vi "test_TCP_TCP Write.vi"(8 "error in (no error)":errorcluster, 11 "TestCase in":refnum<class "Ethernet Protocol Tests.lvclass">) -> (0 "error out":errorcluster, 3 "TestCase out":refnum<class "Ethernet Protocol Tests.lvclass">)   [LabVIEW 2019, in "Ethernet Protocol Tests.lvclass"]
uses:
  Ethernet Protocol Tests.lvclass
  Listener/Listener.lvclass
  Listener/ListenerClassControls/Operation.ctl
  TCP/TCP.lvclass
  D:/GitRepository/niveristand-instrument-addon-classes/Source/Protocols/Protocol Parent/Protocol Parent.lvclass
  TCP/TCP.lvclass/TCP.ctl
  <vilib>/addons/_JKI Toolkits/VI Tester/TestCase.llb/TestCase.lvclass
  C:/Program Files (x86)/National Instruments/LabVIEW 2019/vi.lib/addons/_JKI Toolkits/VI Tester/TestCase.llb/TestCase.lvclass
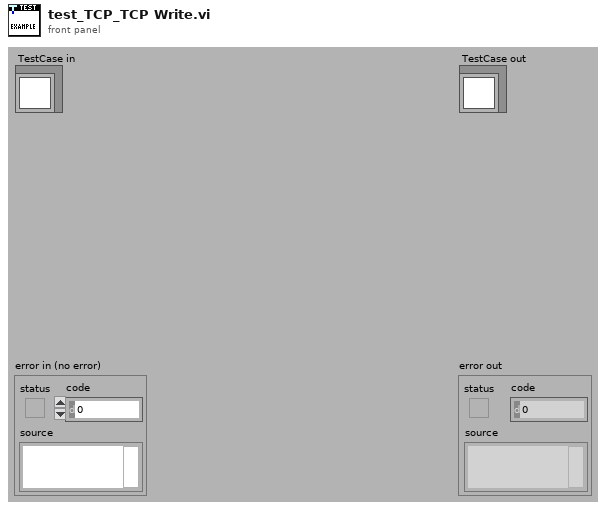
[diagram p1: front panel]
types:
  T1 = typedef "Listener.lvclass/Operation.ctl" = enum16{"Read", "Write"}
  T2 = typedef "Listener.lvclass/TCP Data Structure.ctl" = cluster{"TCP|IP connection ID":refnum<k5>, "IP Address":string, "Port":u16, "Data":string}
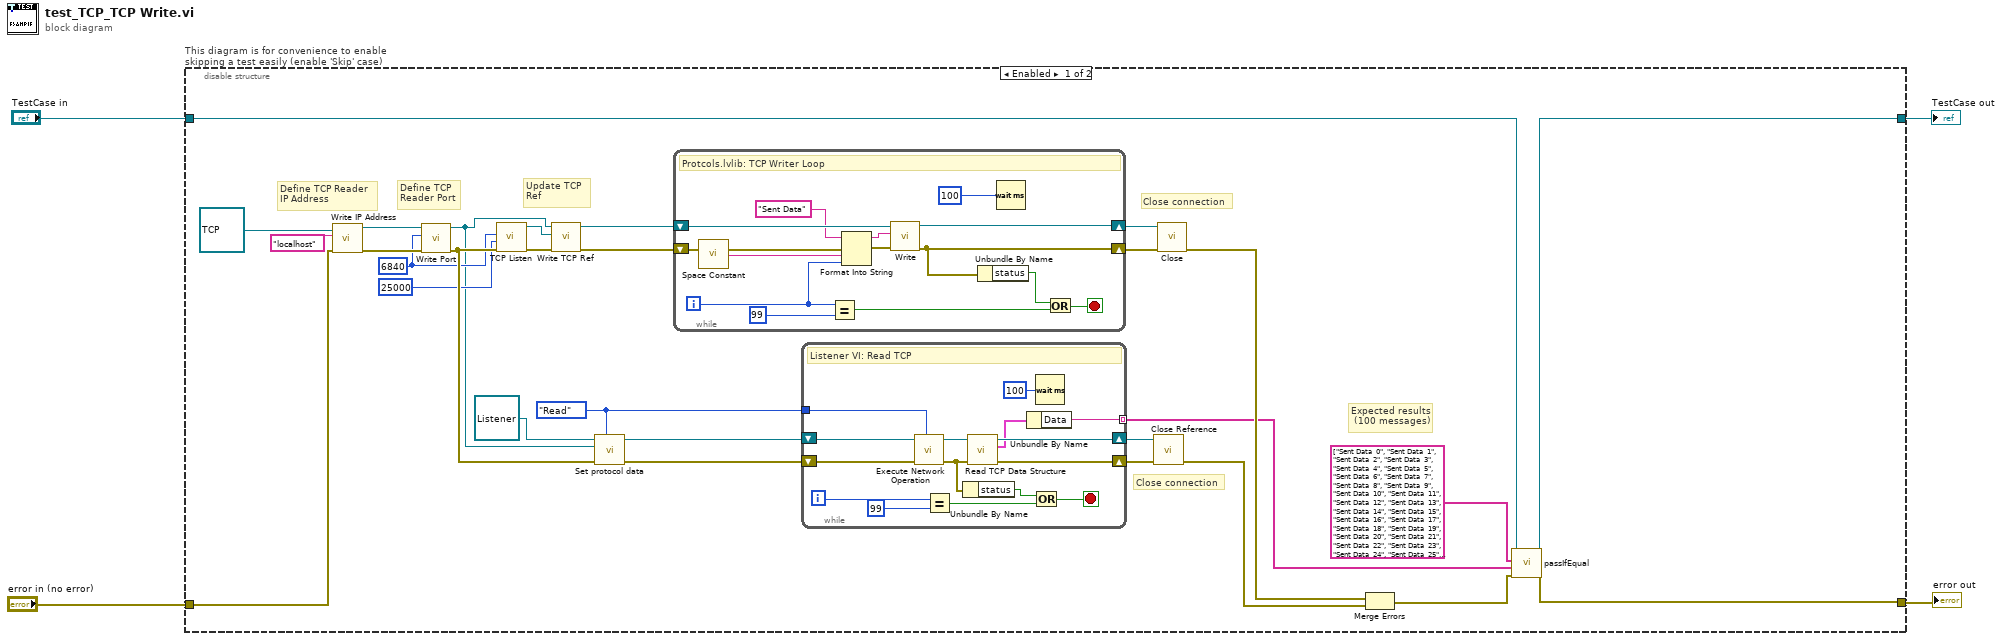
[diagram p0: block diagram]
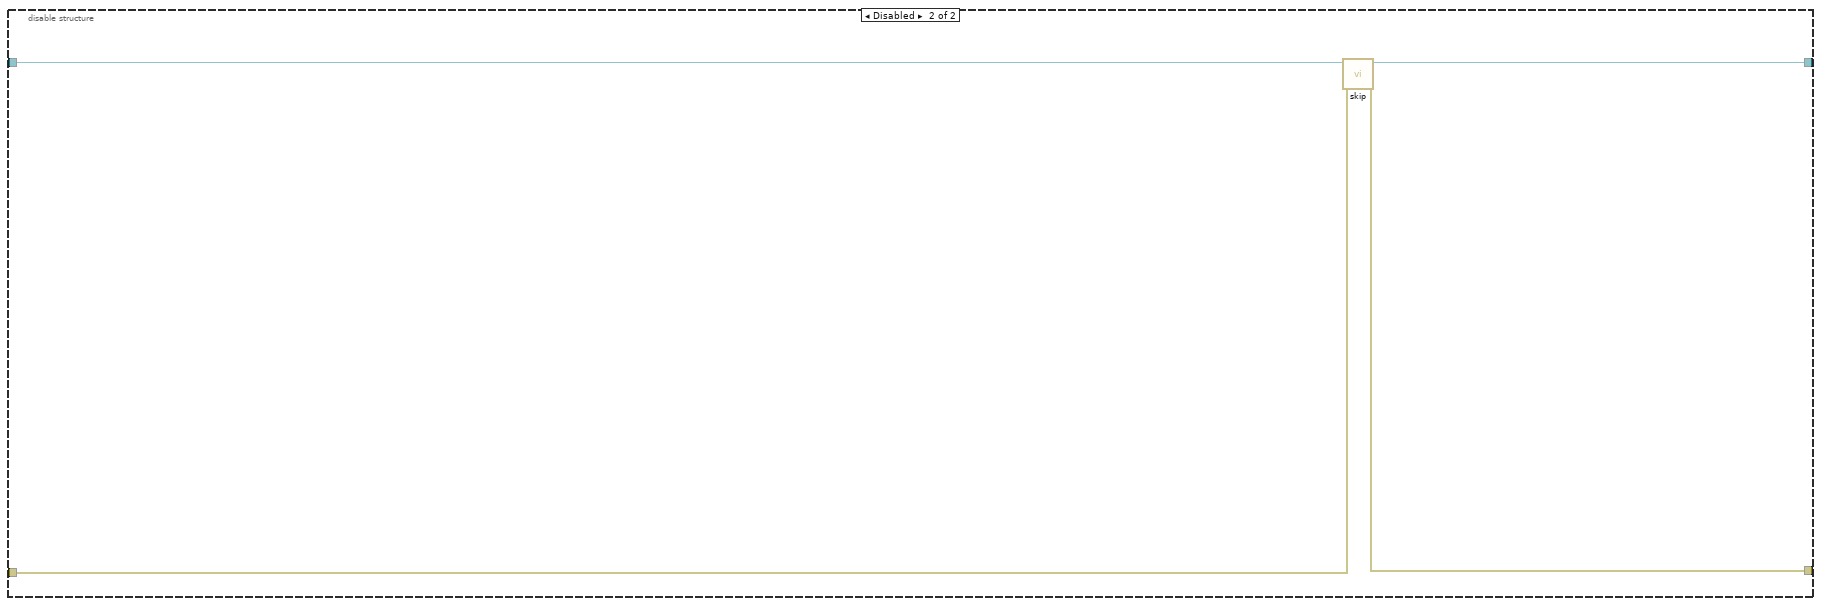
[diagram p2: hidden frame]
diagram:
  n1 = disable-structure "This diagram is for convenience to enable skipping a test easily (enable 'Skip' case)" shown="Enabled" {
    disable-tunnel: "TestCase in" -> [w33 w66]
    disable-tunnel: [w32 w64] -> w1
    disable-tunnel: [w31 w65] -> w3
    disable-tunnel: "error in (no error)" -> [w27 w63]
    frame Enabled {
      w14 = Operation."Read" ("Operation")
      w21 = u16 6840 ("Port")
      # "Close connection"
      # "Close connection"
      # "Update TCP \nRef"
      # "Expected results\n (100 messages)"
      # "Define TCP \nReader Port"
      # "Define TCP Reader \nIP Address"
      n2 = call "Write IP Address.vi"("error in (no error)"=w27, "IP Address"="localhost", "Ethernet in"=refnum<class "TCP.lvclass"> refnum ("Protocols.lvlib:TCP.lvclass")) -> ("error out"=w28:errorcluster, "Ethernet out"=w29:refnum<class "TCP.lvclass">)  [unwired: 7 in]
      n3 = call "Write Port.vi"("error in (no error)"=w28, "Port"=w21, "Ethernet in"=w29) -> ("error out"=w22:errorcluster, "Ethernet out"=w16:refnum<class "TCP.lvclass">)  [unwired: 7 in]
      n4 = call <vilib>:"TCP Listen.vi"("error in (no error)"=w22, "timeout ms (wait forever: -1)"=25000, "port"=w21) -> ("error out"=w19:errorcluster, "connection ID"=w15:refnum<k5>)  [unwired: 4 in, 3 out]
      n5 = call "Write TCP Ref.vi"("error in (no error)"=w19, "TCP Ref"=w15, "Ethernet in"=w16) -> ("error out"=w18:errorcluster, "Ethernet out"=w17:refnum<class "TCP.lvclass">)  [unwired: 7 in]
      n6 = call "Set protocol data.vi"("Operation"=w14, "error in (no error)"=w22, "Protocols.lvlib:Protocol Parent.lvclass"=w16, "Listener In.lvclass"=refnum<class "Listener.lvclass"> refnum ("Listener.lvclass")) -> ("error out"=w23:errorcluster, "Listener Out.lvclass"=w24:refnum<class "Listener.lvclass">)  [unwired: 6 in]
      n7 = while {
        shift-right: [w58] -> w10
        shift-left: w18 -> [w54]
        shift-right: [w57] -> w9
        shift-left: w17 -> [w59]
        i -> [w49]
        stop <- w61 stop-if-true
        # "Protcols.lvlib: TCP Writer Loop"
        n8 = call <vilib>:"Space Constant.vi"() -> ("String"=w53:string)
        n9 = Equal?(x=w49, y=99 ("x")) -> (x = y?=w62:bool)
        n10 = Format Into String(initial string="Sent Data" ("String"), error in=w54, w53, w49) -> (resulting string=w51:string, error out=w52:errorcluster)  [unwired: 1 in]
        n11 = call-dynamic "Write.vi"("error in (no error)"=w52, "String"=w51, "Ethernet in"=w59) -> ("error out"=w58:errorcluster, "Ethernet out"=w57:refnum<class "TCP.lvclass">)  [unwired: 7 in]
        n12 = Unbundle By Name(w58) -> ("status"=w56:bool)
        n13 = Wait (ms)(milliseconds to wait=u32 100) -> ()  [unwired: 1 out]
        n14 = Or(x=w56, y=w62) -> (x .or. y?=w61:bool)
      }
      n15 = while {
        shift-right: [w35] -> w12
        shift-left: w23 -> [w48]
        shift-right: [w36] -> w13
        shift-left: w24 -> [w47]
        tunnel: w14 -> [w42]
        tunnel: [w41] -> w7 mode=indexing
        i -> [w40]
        stop <- w45 stop-if-true
        # "Listener VI: Read TCP"
        n16 = call "Execute Network Operation.vi"("Operation"=w42, "error in (no error)"=w48, "Listener In.lvclass"=w47) -> ("error out"=w38:errorcluster, "Listener Out.lvclass"=w37:refnum<class "Listener.lvclass">)  [unwired: 7 in]
        n17 = Equal?(x=w40, y=99 ("x")) -> (x = y?=w44:bool)
        n18 = Unbundle By Name(w38) -> ("status"=w46:bool)
        n19 = call-dynamic "Read TCP Data Structure.vi"("error in (no error)"=w38, "Listener in"=w37) -> ("error out"=w35:errorcluster, "TCP|IP Data Structure"=w34:T2, "Listener out"=w36:refnum<class "Listener.lvclass">)  [unwired: 7 in]
        n20 = Unbundle By Name(w34) -> ("Data"=w41:string)
        n21 = Or(x=w46, y=w44) -> (x .or. y?=w45:bool)
        n22 = Wait (ms)(milliseconds to wait=u32 100) -> ()  [unwired: 1 out]
      }
      n23 = call "Close Reference.vi"("error in (no error)"=w12, "Listener In.lvclass"=w13) -> ("error out"=w11:errorcluster)  [unwired: 9 in]
      n24 = call-dynamic "Close.vi"("error in (no error)"=w10, "Ethernet in"=w9) -> ("error out"=w8:errorcluster)  [unwired: 8 in, 1 out]
      n25 = Merge Errors(w8, w11) -> (w26:errorcluster)
      n26 = call-dynamic "passIfEqual.vi"("error in (no error)"=w26, "y"=w7, "x"=string[] ["Sent Data  0", "Sent Data  1", "Sent Data  2", "Sent Data  3", "Sent Data  4", "Sent Data  5", "Sent Data  6", "Sent Data  7", "Sent Data  8", "Sent Data  9", "Sent Data  10", "Sent Data  11", "Sent Data  12", "Sent Data  13", "Sent Data  14", "Sent Data  15", "Sent Data  16", "Sent Data  17", "Sent Data  18", "Sent Data  19", "Sent Data  20", "Sent Data  21", "Sent Data  22", "Sent Data  23", "Sent Data  24", "Sent Data  25", "Sent Data  26", "Sent Data  27", "Sent Data  28", "Sent Data  29", "Sent Data  30", "Sent Data  31", "Sent Data  32", "Sent Data  33", "Sent Data  34", "Sent Data  35", "Sent Data  36", "Sent Data  37", "Sent Data  38", "Sent Data  39", "Sent Data  40", "Sent Data  41", "Sent Data  42", "Sent Data  43", "Sent Data  44", "Sent Data  45", "Sent Data  46", "Sent Data  47", "Sent Data  48", "Sent Data  49", "Sent Data  50", "Sent Data  51", "Sent Data  52", "Sent Data  53", "Sent Data  54", "Sent Data  55", "Sent Data  56", "Sent Data  57", "Sent Data  58", "Sent Data  59", "Sent Data  60", "Sent Data  61", "Sent Data  62", "Sent Data  63", "Sent Data  64", "Sent Data  65", "Sent Data  66", "Sent Data  67", "Sent Data  68", "Sent Data  69", "Sent Data  70", "Sent Data  71", "Sent Data  72", "Sent Data  73", "Sent Data  74", "Sent Data  75", "Sent Data  76", "Sent Data  77", "Sent Data  78", "Sent Data  79", "Sent Data  80", "Sent Data  81", "Sent Data  82", "Sent Data  83", "Sent Data  84", "Sent Data  85", "Sent Data  86", "Sent Data  87", "Sent Data  88", "Sent Data  89", "Sent Data  90", "Sent Data  91", "Sent Data  92", "Sent Data  93", "Sent Data  94", "Sent Data  95", "Sent Data  96", "Sent Data  97", "Sent Data  98", "Sent Data  99"] ("Array"), "TestCase in"=w33) -> ("error out"=w31:errorcluster, "TestCase out"=w32:refnum<class "Ethernet Protocol Tests.lvclass">)  [unwired: 6 in]
    }
    frame Disabled {
      # "skip test result while test is under development"
      n27 = call <vilib>:"skip.vi"("error in (no error)"=w63, "TestCase in"=w66) -> ("error out"=w65:errorcluster, "TestCase out"=w64:refnum<class "Ethernet Protocol Tests.lvclass">)  [unwired: 8 in]
    }
  }
  "error out" <- w3
  "TestCase out" <- w1
